vi "Move Sequence.vi"(8 "Distance Up":dbl=28.0, 11 "Distance Down":dbl=28.0) -> ()   [LabVIEW 2014]
uses:
  Begin/Global Variables.vi
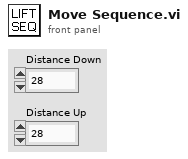
[diagram p1: front panel]
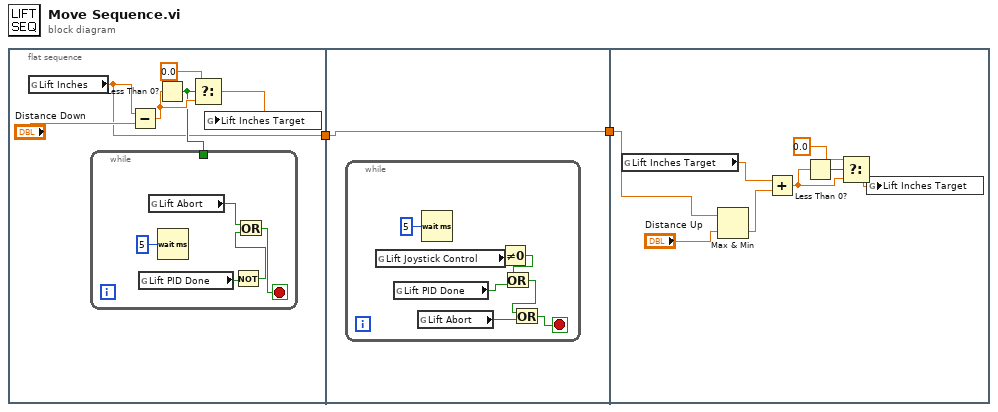
[diagram p0: block diagram]
diagram:
  n1 = flat-sequence {
    tunnel: [w3] -> w1
    tunnel: [w14] -> w2
    tunnel: w1 -> [w14]
    tunnel: w2 -> [w22]
    frame #0 {
      n2 = global read "Global Variables.vi" "Lift Inches"() -> (w3:dbl)
      n3 = Subtract(x=w3, y="Distance Down") -> (x-y=w7:dbl)
      n4 = Less Than 0?(x=w7) -> (x < 0?=w4:bool)
      n5 = while {
        tunnel: w4 -> [_]
        stop <- w12 stop-if-true
        n6 = global read "Global Variables.vi" "Lift PID Done"() -> (w10:bool)
        n7 = global read "Global Variables.vi" "Lift Abort"() -> (w11:bool)
        n8 = Wait (ms)(milliseconds to wait=u32 5) -> ()  [unwired: 1 out]
        n9 = Not(x=w10) -> (.not. x?=w9:bool)
        n10 = Or(x=w11, y=w9) -> (x .or. y?=w12:bool)
      }
      n11 = Select(t=0.0, s=w4, f=w7) -> (s? t:f=w6:dbl)
      n12 = global write "Global Variables.vi" "Lift Inches Target"(w6) -> ()
    }
    frame #1 {
      n13 = while {
        stop <- w17 stop-if-true
        n14 = global read "Global Variables.vi" "Lift Joystick Control"() -> (w19:dbl)
        n15 = global read "Global Variables.vi" "Lift PID Done"() -> (w20:bool)
        n16 = global read "Global Variables.vi" "Lift Abort"() -> (w15:bool)
        n17 = Wait (ms)(milliseconds to wait=u32 5) -> ()  [unwired: 1 out]
        n18 = Not Equal To 0?(x=w19) -> (x != 0?=w18:bool)
        n19 = Or(x=w18, y=w20) -> (x .or. y?=w16:bool)
        n20 = Or(x=w16, y=w15) -> (x .or. y?=w17:bool)
      }
    }
    frame #2 {
      n21 = global read "Global Variables.vi" "Lift Inches Target"() -> (w27:dbl)
      n22 = Max & Min(x=w22, y="Distance Up") -> (min(x,y)=w23:dbl)  [unwired: 1 out]
      n23 = Add(x=w27, y=w23) -> (x+y=w28:dbl)
      n24 = Less Than 0?(x=w28) -> (x < 0?=w29:bool)
      n25 = Select(t=0.0, s=w29, f=w28) -> (s? t:f=w26:dbl)
      n26 = global write "Global Variables.vi" "Lift Inches Target"(w26) -> ()
    }
  }
